vi "Axis data to Arr (SubVI).vi"(0 "new X element":dbl, 5 "new Y element":dbl, 7 "new Z element":dbl, 11 "error in":errorcluster, 12 "X Arr in":dbl[](array[numeric]), 13 "Y Arr in":dbl[](array[numeric]), 14 "Z Arr in":dbl[](array[numeric])) -> (4 "X Arr Out":dbl[](array[numeric]), 6 "Y Arr Out":dbl[](array[numeric]), 8 "Z Arr Out":dbl[](array[numeric]), 15 "error out":errorcluster)   [LabVIEW 2013]
doc: "Сохранение текущего измерения МП оси в массив.."
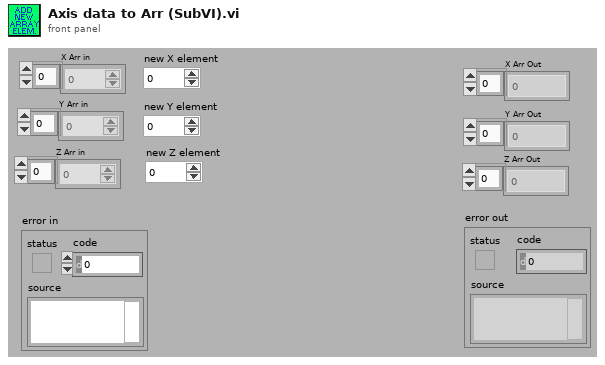
[diagram p1: front panel]
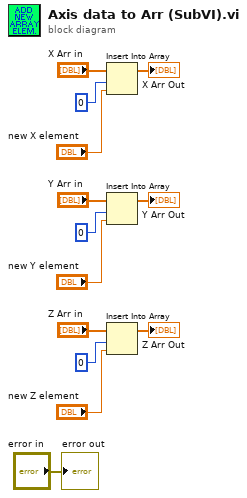
[diagram p0: block diagram]
diagram:
  n1 = Insert Into Array(array="X Arr in", index=0, new element="new X element") -> (→"X Arr Out":dbl[])
  n2 = Insert Into Array(array="Y Arr in", index=0, new element="new Y element") -> (→"Y Arr Out":dbl[])
  n3 = Insert Into Array(array="Z Arr in", index=0, new element="new Z element") -> (→"Z Arr Out":dbl[])
  "error out" <- "error in"
